vi "_2_deleteemptyarray2.vi"(1 "input":string[](array[string])) -> (0 "in_cons":string[](array[string]))   [LabVIEW 2011]
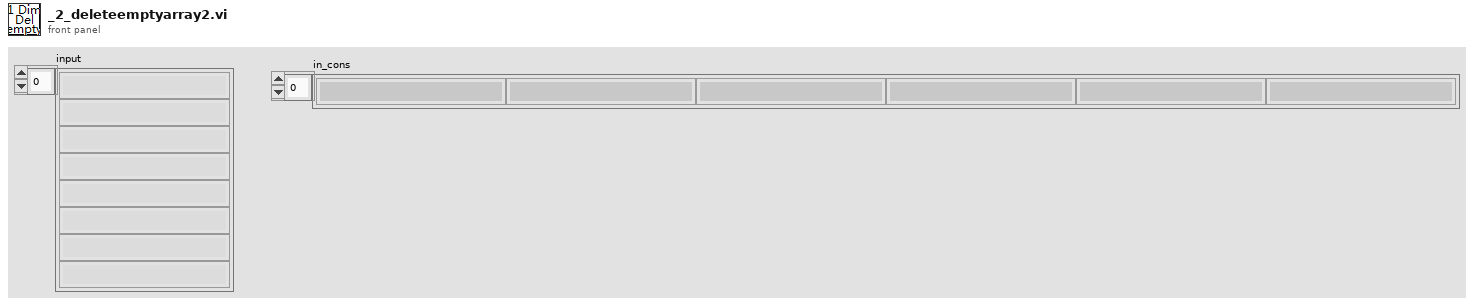
[diagram p1: front panel]
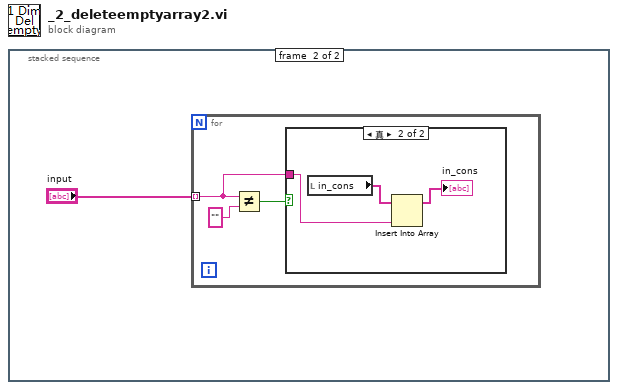
[diagram p0: block diagram]
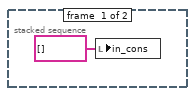
[diagram p2: hidden frame]
diagram:
  n1 = stacked-sequence {
    frame #0 {
      n2 = local write "in_cons"(string[] [] ("in_cons")) -> ()
    }
    frame #1 {
      n3 = for {
        tunnel: "input" -> [w3] mode=indexing
        n4 = Not Equal?(x=w3, y="") -> (x != y?=w4:bool)
        n5 = case shown="真" w4 {
          tunnel: w3 -> [_ w8]
          frame False {
          }
          frame True {
            n6 = local read "in_cons"() -> (w7:string[])
            n7 = Insert Into Array(array=w7, new element=w8) -> (→"in_cons":string[])  [unwired: 1 in]
          }
        }
      }
    }
  }
